vi "HTTP PATCH.vi"(6 "request specific headers":T1[](array[typedef]), 7 "timeout (0 = Use Default)":i32, 8 "error in (no error)":errorcluster, 9 "Request body":string, 10 "Path":string, 11 "REST Client in":refnum<class "REST Client.lvclass">) -> (0 "error out":errorcluster, 1 "Response body":string, 2 "Response Header":refnum<class "Response Headers.lvclass">, 3 "REST Client out":refnum<class "REST Client.lvclass">)   [LabVIEW 2020, in "REST Client.lvlib" / "REST Client.lvclass"]
doc: "Perform a HTTP POST request.\n\nThe VI provides multiple arguments for defining how to perform the HTTP request.\n\n<b>Path</b> specifies the path beneath the Base URL to be used for the HTTP request.\n\n<b>Request body</b> specifies the body of the request to be send to the server.\n\n<b>request specific headers</b> specifies an array of headers to be used with this particular HTTP request. The Default Headers specified upon creation of the JKI REST Client together with the request specific headers will all be used for the HTTP request."
uses:
  REST Client.lvclass
  HTTP Header.ctl
  Response Headers/Response Headers.lvclass
  HTTP Methods.ctl
  response/response.lvclass
  REST Client.lvclass/REST Client.ctl
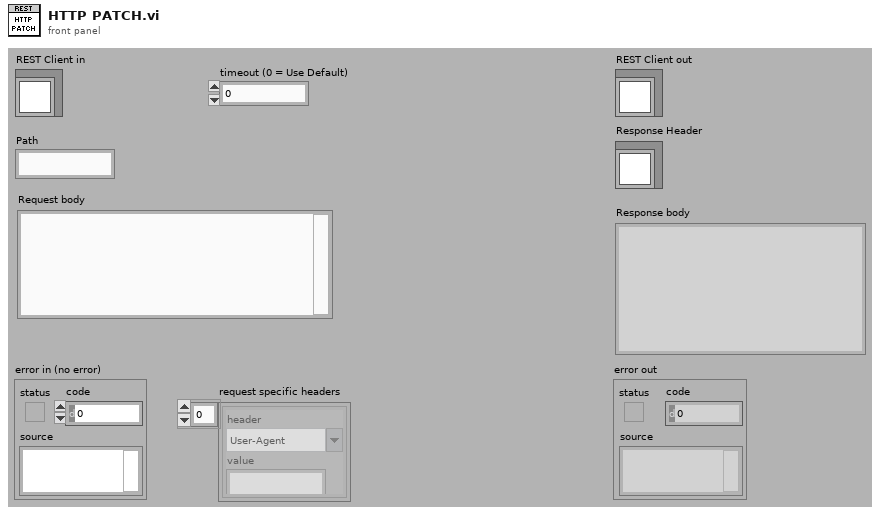
[diagram p1: front panel]
types:
  T1 = typedef "REST Client.lvlib/REST Client.lvclass/HTTP Header.ctl" = cluster{"header":string, "value":string}
  T2 = typedef "REST Client.lvlib/REST Client.lvclass/HTTP Methods.ctl" = enum16{"GET", "HEAD", "POST", "PUT", "DELETE", "PATCH"}
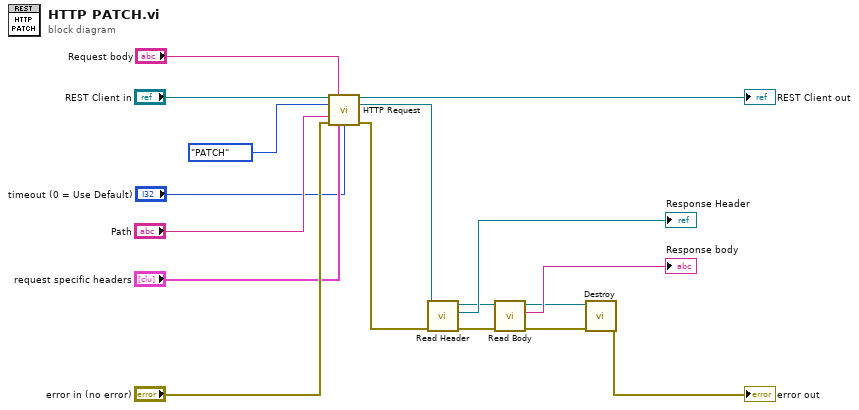
[diagram p0: block diagram]
diagram:
  n1 = call-dynamic "HTTP Request.vi"("REST Client in"="REST Client in", "Request body"="Request body", "Method"=HTTP_Methods."PATCH", "Path"="Path", "error in (no error)"="error in (no error)", "request specific headers"="request specific headers", "timeout (0 = Use Default)"="timeout (0 = Use Default)") -> ("REST Client out"=→"REST Client out":refnum<class "REST Client.lvclass">, "response"=w3:refnum<class "response.lvclass">, "error out"=w2:errorcluster)  [unwired: 6 in]
  n2 = call-dynamic "Read Header.vi"("error in (no error)"=w2, "response in"=w3) -> ("error out"=w7:errorcluster, "Header"=→"Response Header":refnum<class "Response Headers.lvclass">, "response out"=w6:refnum<class "response.lvclass">)  [unwired: 7 in]
  n3 = call-dynamic "Read Body.vi"("error in (no error)"=w7, "response in"=w6) -> ("error out"=w4:errorcluster, "body"=→"Response body":string, "response out"=w5:refnum<class "response.lvclass">)  [unwired: 7 in]
  n4 = call-dynamic "Destroy.vi"("error in (no error)"=w4, "response in"=w5) -> ("error out"=→"error out":errorcluster)  [unwired: 9 in]
